vi "ConvertGaussianParameters.vi"(0 "Best Fits":dbl[](array[numeric]), 1 "Subsampling":u16(ring)=16 items=["1"=1, "2"=2, "4"=4, "8"=8, "16"=16], 2 "Pixel Size":cluster{"X Step":sgl, "Y Step":sgl}={"X Step"=1.0, "Y Step"=1.0} {"Y Step" format="%.2f"; "X Step" format="%.2f"}, 3 "ROIOffsetX":dbl, 4 "ROIOffsetY":dbl) -> (5 "output cluster":T1)   [LabVIEW 2015]
panel:
  # "x"
  # "µm"
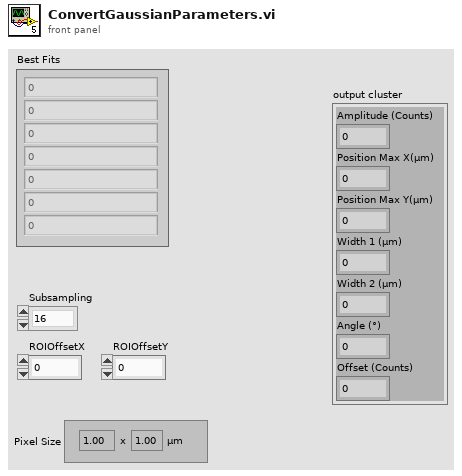
[diagram p1: front panel]
types:
  T1 = cluster{"Amplitude (Counts)":dbl, "Position Max X(µm)":dbl, "Position Max Y(µm)":dbl, "Width 1 (µm)":dbl, "Width 2 (µm)":dbl, "Angle (°)":dbl, "Offset (Counts)":dbl}
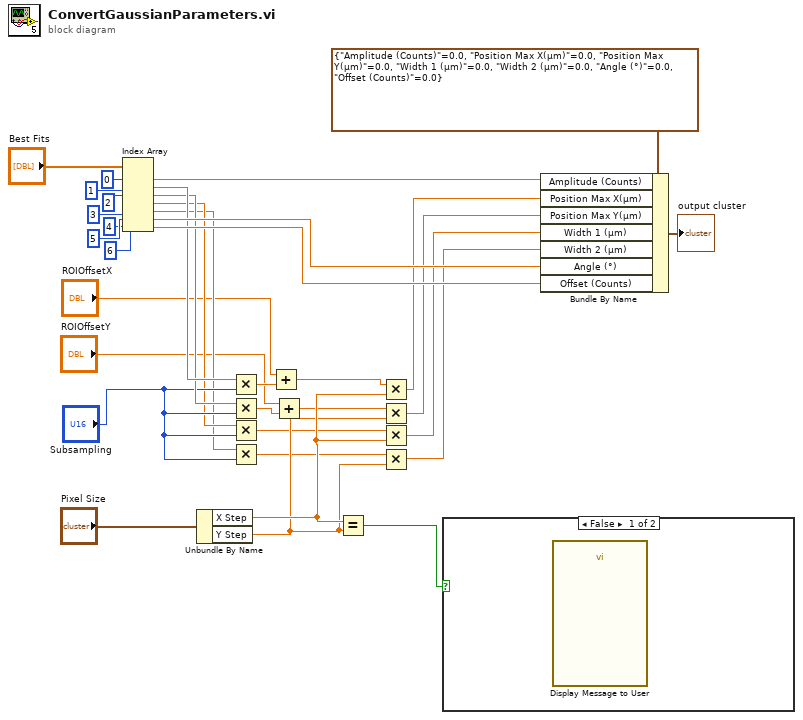
[diagram p0: block diagram]
diagram:
  n1 = Index Array(array="Best Fits", index #1=0 ("index"), index #2=1 ("index"), index #3=2 ("index"), index #4=3 ("index"), index #5=4 ("index"), index #6=5 ("index"), index #7=6 ("index")) -> (element #1=w26:dbl, element #2=w15:dbl, element #3=w14:dbl, element #4=w12:dbl, element #5=w11:dbl, element #6=w25:dbl, element #7=w24:dbl)
  n2 = Unbundle By Name("Pixel Size") -> ("X Step"=w17:sgl, "Y Step"=w16:sgl)
  n3 = Multiply(x=w15, y="Subsampling") -> (x*y=w8:dbl)
  n4 = Multiply(x=w14, y="Subsampling") -> (x*y=w7:dbl)
  n5 = Multiply(x=w12, y="Subsampling") -> (x*y=w10:dbl)
  n6 = Multiply(x=w11, y="Subsampling") -> (x*y=w9:dbl)
  n7 = Add(x="ROIOffsetX", y=w8) -> (x+y=w5:dbl)
  n8 = Add(x="ROIOffsetY", y=w7) -> (x+y=w6:dbl)
  n9 = Equal?(x=w17, y=w16) -> (x = y?=w22:bool)
  n10 = Multiply(x=w5, y=w17) -> (x*y=w21:dbl)
  n11 = Multiply(x=w6, y=w16) -> (x*y=w20:dbl)
  n12 = Multiply(x=w10, y=w17) -> (x*y=w19:dbl)
  n13 = Multiply(x=w9, y=w16) -> (x*y=w18:dbl)
  n14 = case shown="False" w22 {
    frame False {
      n15 = call "Display Message to User"() -> ()  [unwired: 10 in, 2 out]
    }
    frame True {
    }
  }
  n16 = Bundle By Name(cluster=T1 {"Amplitude (Counts)"=0.0, "Position Max X(µm)"=0.0, "Position Max Y(µm)"=0.0, "Width 1 (µm)"=0.0, "Width 2 (µm)"=0.0, "Angle (°)"=0.0, "Offset (Counts)"=0.0} ("input cluster"), "Amplitude (Counts)"=w26, "Position Max X(µm)"=w21, "Position Max Y(µm)"=w20, "Width 1 (µm)"=w19, "Width 2 (µm)"=w18, "Angle (°)"=w25, "Offset (Counts)"=w24) -> (→"output cluster":T1)
